vi "FGVScannerConfig.vi"(7 "Enum":T1, 8 "error in":errorcluster, 9 "scannerTimeConstantIn":u16, 10 "scannerIdIn":i8) -> (0 "error out":errorcluster, 1 "scannerTimeConstantOut":u16, 2 "scannerIdOut":i8)   [LabVIEW 2016]
uses:
  controls/Enum.ctl
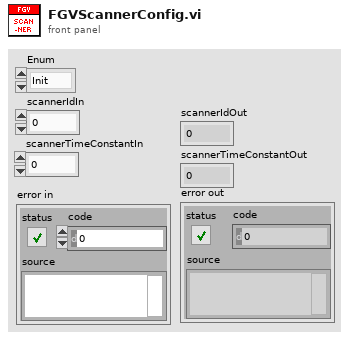
[diagram p1: front panel]
types:
  T1 = typedef "Enum.ctl" = enum16{"Init", "Read", "Write"}
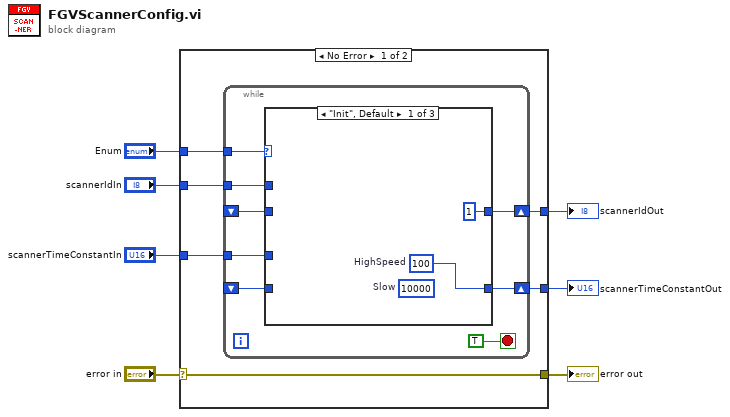
[diagram p0: block diagram]
diagram:
  n1 = case shown="No Error" "error in" {
    selector: "error in" -> [w13 w30]
    tunnel: [w13 w30] -> w6
    tunnel: "Enum" -> [w12 _]
    tunnel: "scannerIdIn" -> [w11 w29]
    tunnel: [w10 w29] -> w3
    tunnel: "scannerTimeConstantIn" -> [w9 w28]
    tunnel: [w8 w28] -> w1
    frame No Error {
      n2 = while {
        tunnel: w12 -> [w21]
        tunnel: w11 -> [w20]
        shift-right: [w19] -> w10
        shift-left: _ -> [w18]
        tunnel: w9 -> [w17]
        shift-right: [w16] -> w8
        shift-left: _ -> [w15]
        stop <- TRUE stop-if-true
        n3 = case shown="\"Init\", Default" w21 {
          tunnel: w20 -> [_ _ w27]
          tunnel: [i8 1 ("scannerIdIn") w25 w27] -> w19
          tunnel: w18 -> [_ w25 _]
          tunnel: w17 -> [_ _ w26]
          tunnel: [w22 w24 w26] -> w16
          tunnel: w15 -> [_ w24 _]
          frame "Init", Default {
            w22 = u16 100  # HighSpeed
            (unwired) u16 10000  # Slow
          }
          frame "Read" {
          }
          frame "Write" {
          }
        }
      }
    }
    frame Error {
    }
  }
  "error out" <- w6
  "scannerIdOut" <- w3
  "scannerTimeConstantOut" <- w1
